vi "Mapping.vi"(11 "Relation in":refnum<class "Relation.lvclass">) -> (2 "Mapping":T1=enum."OneToMany")   [LabVIEW 2020, in "Conditu2.lvlib" / "Columns.lvlib" / "Relation.lvclass"]
uses:
  Relation.lvclass
  Relation Mapping.ctl
  Relation.lvclass/Relation.ctl
  Conditu2.lvlib
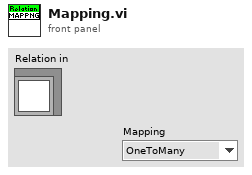
[diagram p1: front panel]
types:
  T1 = typedef "Conditu2.lvlib/Relation Mapping.ctl" = enum16{"OneToOne", "OneToMany", "ManyToOne", "ManyToMany"}
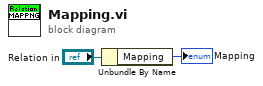
[diagram p0: block diagram]
diagram:
  n1 = Unbundle By Name("Relation in") -> ("Mapping"=→"Mapping":T1)
